vi "Delete Sample Offset DVR.vi"(8 "error in (no error)":errorcluster, 11 "Waveform Session in":refnum<class "Waveform Session.lvclass">) -> (0 "error out":errorcluster, 3 "Waveform Session out":refnum<class "Waveform Session.lvclass">)   [LabVIEW 2020, in "NI_VS Custom Device Waveform API.lvlib" / "Waveform Session.lvclass"]
uses:
  Waveform Session.lvclass
  Waveform Session.lvclass/Waveform Session.ctl
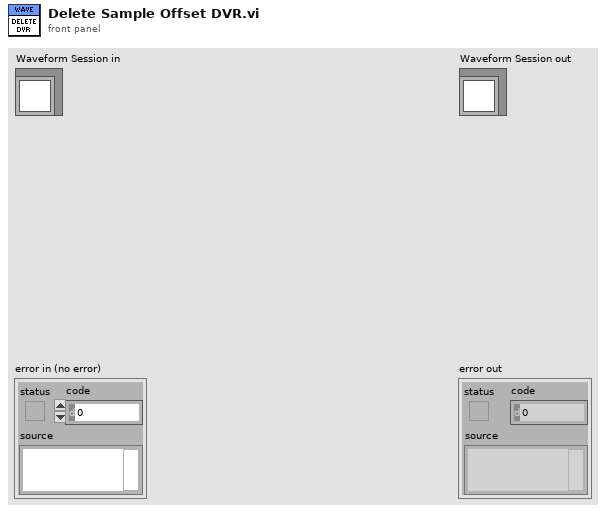
[diagram p1: front panel]
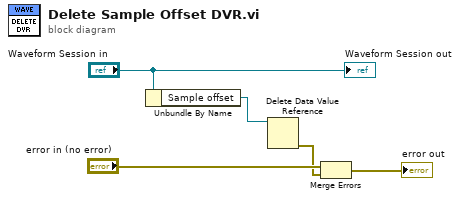
[diagram p0: block diagram]
diagram:
  n1 = Unbundle By Name("Waveform Session in") -> ("Sample offset"=w4:refnum<data-value>)
  n2 = Delete Data Value Reference(data value reference=w4) -> (error out=w2:errorcluster)  [unwired: 1 in, 1 out]
  n3 = Merge Errors("error in (no error)", w2) -> (→"error out":errorcluster)
  "Waveform Session out" <- "Waveform Session in"
